vi "casestructures.vi"() -> ()   [LabVIEW 2025]
panel:
  in  "Enter a String (Case Insensitive!)":string
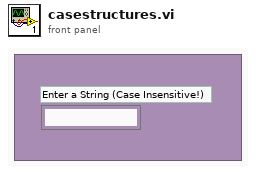
[diagram p1: front panel]
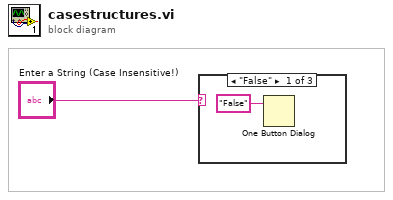
[diagram p0: block diagram]
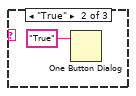
[diagram p2: hidden frame]
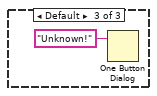
[diagram p3: hidden frame]
diagram:
  n1 = case shown="\"False\"" "Enter a String (Case Insensitive!)" {
    frame "False" {
      n2 = One Button Dialog(message="False") -> ()  [unwired: 1 in, 1 out]
    }
    frame "True" {
      n3 = One Button Dialog(message="True") -> ()  [unwired: 1 in, 1 out]
    }
    frame Default {
      n4 = One Button Dialog(message="Unknown!") -> ()  [unwired: 1 in, 1 out]
    }
  }
